vi "State Change Core.vi"(8 "error in (no error)":errorcluster, 10 "Transition State":refnum<class "State Change Core.lvclass">, 11 "Context in":refnum<class "Context.lvclass">) -> (0 "error out":errorcluster, 3 "Context out":refnum<class "Context.lvclass">)   [LabVIEW 2021, in "Context.lvlib" / "Context.lvclass"]
uses:
  Context.lvclass
  C:/PPLs/Design-Patterns/State Pattern/State Pattern/State Pattern.lvclass
  State Change Core/State Change Core/State Change Core.lvclass
  Context.lvclass/Context.ctl
  State Pattern/State Pattern.lvclass
  A Context State/A Context State.lvclass
  B Context State/B Context State.lvclass
  C:/PPLs/Design-Patterns/State Pattern/State Change Core/State Change Core/State Change Core.lvclass
  C:/PPLs/Design-Patterns/State Pattern/Context/Context State/Context State.lvclass
  C:/PPLs/Design-Patterns/State Pattern/Context/A Context State/A Context State.lvclass
  C:/PPLs/Design-Patterns/State Pattern/Context/B Context State/B Context State.lvclass
  Context State/Context State.lvclass
  C:/Program Files/National Instruments/LabVIEW 2021/vi.lib/ActorFramework/Actor/Actor.lvclass
  C:/PPLs/Design-Patterns/State Pattern/Context/Context/Context.lvclass
  C:/PPLs/Design-Patterns/State Pattern/xxxx/xxxx/xxxx.lvclass
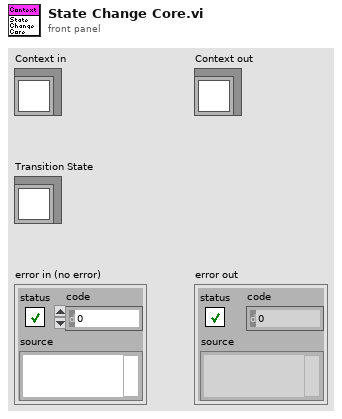
[diagram p1: front panel]
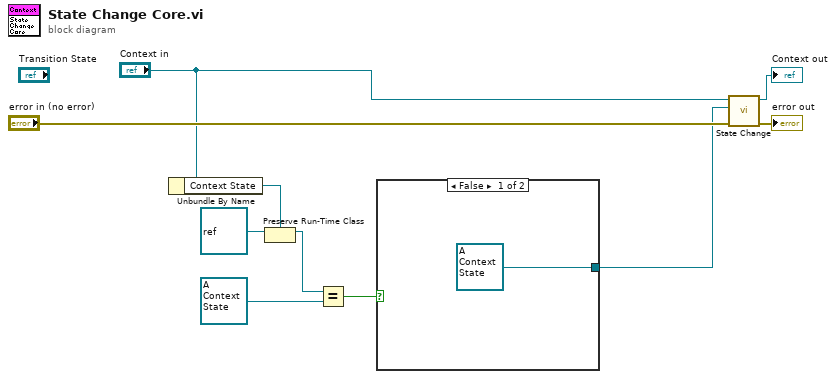
[diagram p0: block diagram]
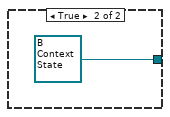
[diagram p2: hidden frame]
diagram:
  n1 = Unbundle By Name("Context in") -> ("Context State"=w5:refnum<class "Context State.lvclass">)
  n2 = Preserve Run-Time Class(object in=refnum<class> refnum ("LabVIEW Object"), 2:w5) -> (object out=w4:refnum<class "Context State.lvclass">)  [unwired: 1 in, 1 out]
  n3 = Equal?(x=w4, y=refnum<class "A Context State.lvclass"> refnum ("Context.lvlib:A Context State.lvclass")) -> (x = y?=w2:bool)
  n4 = case shown="False" w2 {
    tunnel: [refnum<class "A Context State.lvclass"> refnum ("Context.lvlib:A Context State.lvclass") refnum<class "B Context State.lvclass"> refnum ("Context.lvlib:B Context State.lvclass")] -> w1
    frame False {
    }
    frame True {
    }
  }
  n5 = call "State Change.vi"("error in"="error in (no error)", "Transition State"=w1, "State Pattern in"="Context in") -> ("error out"=→"error out":errorcluster, "State Pattern in"=→"Context out":refnum<class "Context.lvclass">)  [unwired: 7 in]
